vi "计算主体.vi"(2 "算法集合":string[][](array[string])=[["a*(b-c/d)"], ["a-(b-c)+d"], ["a-b+c+d"], ["a*(b+c)-d"], ["a-(b-c)*d"], ["a+b/c+d"], ["a+(b/c)*d"], ["a*b*c-d"], ["a*b+c*d"], ["a*(b+c)+d"], ["a+(b-c)*d"], ["(a-b/c)*d"], ["(a*b-c)*d"], ["(a-(b-c))*d"], ["(a-b+c)*d"], ["a+(b*c)+d"], ["a*b-c*d"], ["(a*(b+c))*d"], ["a*(b-c)-d"], ["(a*(b+c))/d"], ["(a-(b+c))*d"], ["a/(b/c)+d"], ["a/(b-(c/d))"], ["a*(b-c)*d"], ["a*(b-c)+d"], ["a+(b-c)+d"], ["a+(b-c)-d"], ["a+(b*c)-d"], ["(a-(b*c))*d"], ["(a-(b/c))*d"], ["a*b-c*d"], ["a*b+c*d"], ["(a+b/c)*d"], ["b*(a-c/d)"], ["b-(a-c)+d"], ["b-a+c+d"], ["b*(a+c)-d"], ["b-(a-c)*d"], ["b+a/c+d"], ["b+(a/c)*d"], ["b*a*c-d"], ["b*a+c*d"], ["b*(a+c)+d"], ["b+(a-c)*d"], ["(b-a/c)*d"], ["(b*a-c)*d"], ["(b-(a-c))*d"], ["(b-a+c)*d"], ["b+(a*c)+d"], ["b*a-c*d"], ["(b*(a+c))*d"], ["b*(a-c)-d"], ["(b*(a+c))/d"], ["(b-(a+c))*d"], ["b/(a/c)+d"], ["b/(a-(c/d))"], ["b*(a-c)*d"], ["b*(a-c)+d"], ["b+(a-c)+d"], ["b+(a-c)-d"], ["b+(a*c)-d"], ["(b-(a*c))*d"], ["(b-(a/c))*d"], ["b*a-c*d"], ["b*a+c*d"], ["(b+a/c)*d"], ["d*(b-c/a)"], ["d-(b-c)+a"], ["d-b+c+a"], ["d*(b+c)-a"], ["d-(b-c)*a"], ["d+b/c+a"], ["d+(b/c)*a"], ["d*b*c-a"], ["d*b+c*a"], ["d*(b+c)+a"], ["d+(b-c)*a"], ["(d-b/c)*a"], ["(d*b-c)*a"], ["(d-(b-c))*a"], ["(d-b+c)*a"], ["d+(b*c)+a"], ["d*b-c*a"], ["(d*(b+c))*a"], ["d*(b-c)-a"], ["(d*(b+c))/a"], ["(d-(b+c))*a"], ["d/(b/c)+a"], ["d/(b-(c/a))"], ["d*(b-c)*a"], ["d*(b-c)+a"], ["d+(b-c)+a"], ["d+(b-c)-a"], ["d+(b*c)-a"], ["(d-(b*c))*a"], ["(d-(b/c))*a"], ["d*b-c*a"], ["d*b+c*a"], ["(d+b/c)*a"], ["c*(b-a/d)"], ["c-(b-a)+d"], ["c-b+a+d"], ["c*(b+a)-d"], ["c-(b-a)*d"], ["c+b/a+d"], ["c+(b/a)*d"], ["c*b*a-d"], ["c*b+a*d"], ["c*(b+a)+d"], ["c+(b-a)*d"], ["(c-b/a)*d"], ["(c*b-a)*d"], ["(c-(b-a))*d"], ["(c-b+a)*d"], ["c+(b*a)+d"], ["c*b-a*d"], ["(c*(b+a))*d"], ["c*(b-a)-d"], ["(c*(b+a))/d"], ["(c-(b+a))*d"], ["c/(b/a)+d"], ["c/(b-(a/d))"], ["c*(b-a)*d"], ["c*(b-a)+d"], ["c+(b-a)+d"], ["c+(b-a)-d"], ["c+(b*a)-d"], ["(c-(b*a))*d"], ["(c-(b/a))*d"], ["c*b-a*d"], ["c*b+a*d"], ["(c+b/a)*d"], ["a*(b-d/c)"], ["a-(b-d)+c"], ["a-b+d+c"], ["a*(b+d)-c"], ["a-(b-d)*c"], ["a+b/d+c"], ["a+(b/d)*c"], ["a*b*d-c"], ["a*b+d*c"], ["a*(b+d)+c"], ["a+(b-d)*c"], ["(a-b/d)*c"], ["(a*b-d)*c"], ["(a-(b-d))*c"], ["(a-b+d)*c"], ["a+(b*d)+c"], ["a*b-d*c"], ["(a*(b+d))*c"], ["a*(b-d)-c"], ["(a*(b+d))/c"], ["(a-(b+d))*c"], ["a/(b/d)+c"], ["a/(b-(d/c))"], ["a*(b-d)*c"], ["a*(b-d)+c"], ["a+(b-d)+c"], ["a+(b-d)-c"], ["a+(b*d)-c"], ["(a-(b*d))*c"], ["(a-(b/d))*c"], ["a*b-d*c"], ["a*b+d*c"], ["(a+b/d)*c"], ["a*(d-c/b)"], ["a-(d-c)+b"], ["a-d+c+b"], ["a*(d+c)-b"], ["a-(d-c)*b"], ["a+d/c+b"], ["a+(d/c)*b"], ["a*d*c-b"], ["a*d+c*b"], ["a*(d+c)+b"], ["a+(d-c)*b"], ["(a-d/c)*b"], ["(a*d-c)*b"], ["(a-(d-c))*b"], ["(a-d+c)*b"], ["a+(d*c)+b"], ["a*d-c*b"], ["(a*(d+c))*b"], ["a*(d-c)-b"], ["(a*(d+c))/b"], ["(a-(d+c))*b"], ["a/(d/c)+b"], ["a/(d-(c/b))"], ["a*(d-c)*b"], ["a*(d-c)+b"], ["a+(d-c)+b"], ["a+(d-c)-b"], ["a+(d*c)-b"], ["(a-(d*c))*b"], ["(a-(d/c))*b"], ["a*d-c*b"], ["a*d+c*b"], ["(a+d/c)*b"], ["a*(c-b/d)"], ["a-(c-b)+d"], ["a-c+b+d"], ["a*(c+b)-d"], ["a-(c-b)*d"], ["a+c/b+d"], ["a+(c/b)*d"], ["a*c*b-d"], ["a*c+b*d"], ["a*(c+b)+d"], ["a+(c-b)*d"], ["(a-c/b)*d"], ["(a*c-b)*d"], ["(a-(c-b))*d"], ["(a-c+b)*d"], ["a+(c*b)+d"], ["a*c-b*d"], ["(a*(c+b))*d"], ["a*(c-b)-d"], ["(a*(c+b))/d"], ["(a-(c+b))*d"], ["a/(c/b)+d"], ["a/(c-(b/d))"], ["a*(c-b)*d"], ["a*(c-b)+d"], ["a+(c-b)+d"], ["a+(c-b)-d"], ["a+(c*b)-d"], ["(a-(c*b))*d"], ["(a-(c/b))*d"], ["a*c-b*d"], ["a*c+b*d"], ["(a+c/b)*d"], ["a+b+c+d"], ["a*b*c*d"], ["a*b+c+d"], ["a*b+c-d"], ["a*b-c-d"], ["a*b*c+d"], ["a*b*c-d"], ["a*b+c*d"], ["a*b-c*d"], ["a/b+c+d"], ["a+b-c/d"], ["a*b/c+d"], ["a*b/c-d"], ["a*b/c/d"], ["a*b*c/d"], ["a*b+c/d"], ["a*b-c/d"], ["(a+b)*c+d"], ["(a+b)*c-d"], ["(a-b)*c+d"], ["(a-b)*c-d"], ["(a+b)*c*d"], ["(a-b)*c*d"], ["(a+b)*(c+d)"], ["(a-b)*(c-d)"], ["(a-b)*(c+d)"], ["(a+b+c)*d"], ["(a+b-c)*d"], ["(a-b-c)*d"], ["(a*b+c)*d"], ["(a*b-c)*d"], ["(a-b*c)*d"], ["(a*b-c)/d"], ["(a*b+c)/d"], ["a*b/(c+d)"], ["(a+b)/c+d"], ["(a+b)*c/d"], ["(a-b)*c/d"], ["a*b/(c-d)"], ["(c-a*b)*d"], ["b+a+c+d"], ["b*a*c*d"], ["b*a+c+d"], ["b*a+c-d"], ["b*a-c-d"], ["b*a*c+d"], ["b*a*c-d"], ["b*a+c*d"], ["b*a-c*d"], ["b/a+c+d"], ["b+a-c/d"], ["b*a/c+d"], ["b*a/c-d"], ["b*a/c/d"], ["b*a*c/d"], ["b*a+c/d"], ["b*a-c/d"], ["(b+a)*c+d"], ["(b+a)*c-d"], ["(b-a)*c+d"], ["(b-a)*c-d"], ["(b+a)*c*d"], ["(b-a)*c*d"], ["(b+a)*(c+d)"], ["(b-a)*(c-d)"], ["(b-a)*(c+d)"], ["(b+a+c)*d"], ["(b+a-c)*d"], ["(b-a-c)*d"], ["(b*a+c)*d"], ["(b*a-c)*d"], ["(b-a*c)*d"], ["(b*a-c)/d"], ["(b*a+c)/d"], ["b*a/(c+d)"], ["(b+a)/c+d"], ["(b+a)*c/d"], ["(b-a)*c/d"], ["b*a/(c-d)"], ["(c-b*a)*d"], ["c+b+a+d"], ["c*b*a*d"], ["c*b+a+d"], ["c*b+a-d"], ["c*b-a-d"], ["c*b*a+d"], ["c*b*a-d"], ["c*b+a*d"], ["c*b-a*d"], ["c/b+a+d"], ["c+b-a/d"], ["c*b/a+d"], ["c*b/a-d"], ["c*b/a/d"], ["c*b*a/d"], ["c*b+a/d"], ["c*b-a/d"], ["(c+b)*a+d"], ["(c+b)*a-d"], ["(c-b)*a+d"], ["(c-b)*a-d"], ["(c+b)*a*d"], ["(c-b)*a*d"], ["(c+b)*(a+d)"], ["(c-b)*(a-d)"], ["(c-b)*(a+d)"], ["(c+b+a)*d"], ["(c+b-a)*d"], ["(c-b-a)*d"], ["(c*b+a)*d"], ["(c*b-a)*d"], ["(c-b*a)*d"], ["(c*b-a)/d"], ["(c*b+a)/d"], ["c*b/(a+d)"], ["(c+b)/a+d"], ["(c+b)*a/d"], ["(c-b)*a/d"], ["c*b/(a-d)"], ["(a-c*b)*d"], ["d+b+c+a"], ["d*b*c*a"], ["d*b+c+a"], ["d*b+c-a"], ["d*b-c-a"], ["d*b*c+a"], ["d*b*c-a"], ["d*b+c*a"], ["d*b-c*a"], ["d/b+c+a"], ["d+b-c/a"], ["d*b/c+a"], ["d*b/c-a"], ["d*b/c/a"], ["d*b*c/a"], ["d*b+c/a"], ["d*b-c/a"], ["(d+b)*c+a"], ["(d+b)*c-a"], ["(d-b)*c+a"], ["(d-b)*c-a"], ["(d+b)*c*a"], ["(d-b)*c*a"], ["(d+b)*(c+a)"], ["(d-b)*(c-a)"], ["(d-b)*(c+a)"], ["(d+b+c)*a"], ["(d+b-c)*a"], ["(d-b-c)*a"], ["(d*b+c)*a"], ["(d*b-c)*a"], ["(d-b*c)*a"], ["(d*b-c)/a"], ["(d*b+c)/a"], ["d*b/(c+a)"], ["(d+b)/c+a"], ["(d+b)*c/a"], ["(d-b)*c/a"], ["d*b/(c-a)"], ["(c-d*b)*a"], ["a+c+b+d"], ["a*c*b*d"], ["a*c+b+d"], ["a*c+b-d"], ["a*c-b-d"], ["a*c*b+d"], ["a*c*b-d"], ["a*c+b*d"], ["a*c-b*d"], ["a/c+b+d"], ["a+c-b/d"], ["a*c/b+d"], ["a*c/b-d"], ["a*c/b/d"], ["a*c*b/d"], ["a*c+b/d"], ["a*c-b/d"], ["(a+c)*b+d"], ["(a+c)*b-d"], ["(a-c)*b+d"], ["(a-c)*b-d"], ["(a+c)*b*d"], ["(a-c)*b*d"], ["(a+c)*(b+d)"], ["(a-c)*(b-d)"], ["(a-c)*(b+d)"], ["(a+c+b)*d"], ["(a+c-b)*d"], ["(a-c-b)*d"], ["(a*c+b)*d"], ["(a*c-b)*d"], ["(a-c*b)*d"], ["(a*c-b)/d"], ["(a*c+b)/d"], ["a*c/(b+d)"], ["(a+c)/b+d"], ["(a+c)*b/d"], ["(a-c)*b/d"], ["a*c/(b-d)"], ["(b-a*c)*d"], ["a+d+c+b"], ["a*d*c*b"], ["a*d+c+b"], ["a*d+c-b"], ["a*d-c-b"], ["a*d*c+b"], ["a*d*c-b"], ["a*d+c*b"], ["a*d-c*b"], ["a/d+c+b"], ["a+d-c/b"], ["a*d/c+b"], ["a*d/c-b"], ["a*d/c/b"], ["a*d*c/b"], ["a*d+c/b"], ["a*d-c/b"], ["(a+d)*c+b"], ["(a+d)*c-b"], ["(a-d)*c+b"], ["(a-d)*c-b"], ["(a+d)*c*b"], ["(a-d)*c*b"], ["(a+d)*(c+b)"], ["(a-d)*(c-b)"], ["(a-d)*(c+b)"], ["(a+d+c)*b"], ["(a+d-c)*b"], ["(a-d-c)*b"], ["(a*d+c)*b"], ["(a*d-c)*b"], ["(a-d*c)*b"], ["(a*d-c)/b"], ["(a*d+c)/b"], ["a*d/(c+b)"], ["(a+d)/c+b"], ["(a+d)*c/b"], ["(a-d)*c/b"], ["a*d/(c-b)"], ["(c-a*d)*b"], ["a+b+d+c"], ["a*b*d*c"], ["a*b+d+c"], ["a*b+d-c"], ["a*b-d-c"], ["a*b*d+c"], ["a*b*d-c"], ["a*b+d*c"], ["a*b-d*c"], ["a/b+d+c"], ["a+b-d/c"], ["a*b/d+c"], ["a*b/d-c"], ["a*b/d/c"], ["a*b*d/c"], ["a*b+d/c"], ["a*b-d/c"], ["(a+b)*d+c"], ["(a+b)*d-c"], ["(a-b)*d+c"], ["(a-b)*d-c"], ["(a+b)*d*c"], ["(a-b)*d*c"], ["(a+b)*(d+c)"], ["(a-b)*(d-c)"], ["(a-b)*(d+c)"], ["(a+b+d)*c"], ["(a+b-d)*c"], ["(a-b-d)*c"], ["(a*b+d)*c"], ["(a*b-d)*c"], ["(a-b*d)*c"], ["(a*b-d)/c"], ["(a*b+d)/c"], ["a*b/(d+c)"], ["(a+b)/d+c"], ["(a+b)*d/c"], ["(a-b)*d/c"], ["a*b/(d-c)"], ["(d-a*b)*c"], ["((c-a)*b)*d"], ["((c-a)*d)/b"], ["((c-b)*a)*d"], ["((c-b)*d)/a"], ["((b-a)*c)*d"], ["((b-a)*d)/c"], ["((c-a)*d)*b"], ["((c-a)*b)/d"], ["((a-c)*b)*d"], ["((a-c)*d)/b"], ["((d-a)*b)*c"], ["((d-a)*c)/b"], ["((c-d)*b)*a"], ["((c-d)*a)/b"]], 4 "d":dbl, 5 "c":dbl, 6 "b":dbl, 7 "a":dbl) -> (0 "连接的字符串":string, 1 "算法总数":i32, 3 "所有正解":string[](array[string]))   [LabVIEW 2014]
panel:
  out "算法方程":string[][](array[string]) caption="所有行"
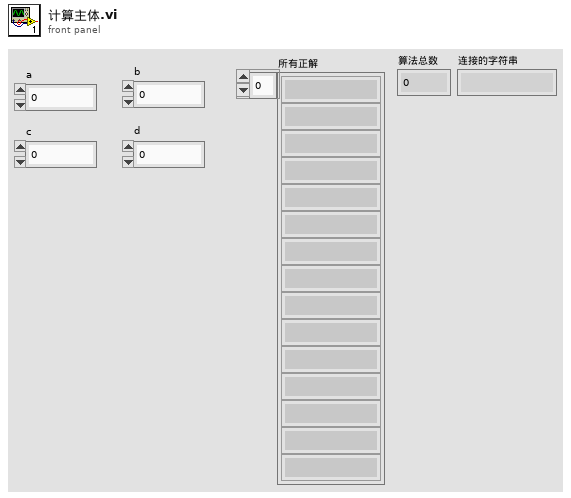
[diagram p1: front panel]
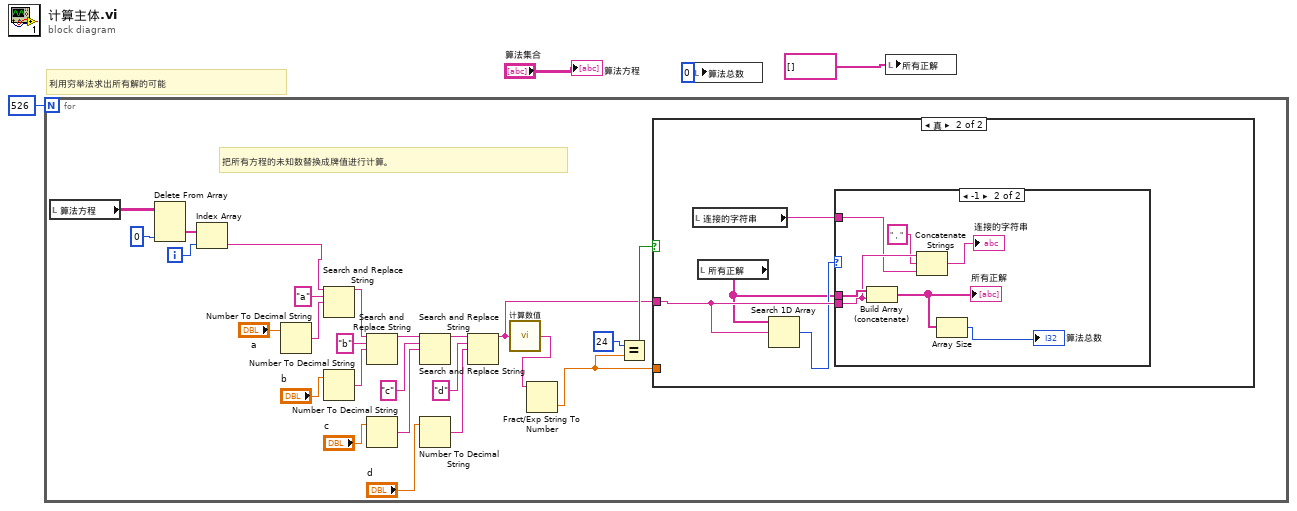
[diagram p0: block diagram]
diagram:
  # "利用穷举法求出所有解的可能"
  n1 = for {
    N: 526 -> [_]
    i -> [w20]
    # "把所有方程的未知数替换成牌值进行计算。"
    n2 = local read "算法方程"() -> (w19:string[][])
    n3 = Delete From Array(array=w19, index (col)=0 ("禁用的索引 (列)")) -> (deleted portion=w21:string[])  [unwired: 2 in, 1 out]
    n4 = Index Array(array=w21, index=w20) -> (element=w7:string)
    n5 = Number To Decimal String(number="a") -> (decimal integer string=w14:string)  [unwired: 1 in]
    n6 = Search and Replace String(input string=w7, search string="a" ("搜索字符串"), replace string=w14) -> (result string=w25:string)  [unwired: 5 in, 3 out]
    n7 = Number To Decimal String(number="b") -> (decimal integer string=w12:string)  [unwired: 1 in]
    n8 = Search and Replace String(input string=w25, search string="b" ("输入字符串"), replace string=w12) -> (result string=w24:string)  [unwired: 5 in, 3 out]
    n9 = Number To Decimal String(number="c") -> (decimal integer string=w10:string)  [unwired: 1 in]
    n10 = Search and Replace String(input string=w24, search string="c" ("输入字符串"), replace string=w10) -> (result string=w23:string)  [unwired: 5 in, 3 out]
    n11 = Number To Decimal String(number="d") -> (decimal integer string=w8:string)  [unwired: 1 in]
    n12 = Search and Replace String(input string=w23, search string="d" ("输入字符串"), replace string=w8) -> (result string=w16:string)  [unwired: 5 in, 3 out]
    n13 = call "计算数值.vi"("表达式"=w16) -> ("结果"=w6:string)
    n14 = Fract/Exp String To Number(string=w6) -> (number=w5:dbl)  [unwired: 3 in, 1 out]
    n15 = Equal?(x=24 ("数字"), y=w5) -> (x = y?=w17:bool)
    n16 = case shown="真" w17 {
      tunnel: w16 -> [_ w33]
      tunnel: w5 -> [_ _]
      frame False {
      }
      frame True {
        n17 = local read "连接的字符串"() -> (w30:string)
        n18 = local read "所有正解"() -> (w31:string[])
        n19 = Search 1D Array(1D array=w31, element=w33) -> (index of element=w32:i32)  [unwired: 1 in]
        n20 = case shown="-1" w32 {
          tunnel: w33 -> [_ w38]
          tunnel: w31 -> [_ w40]
          tunnel: w30 -> [_ w36]
          frame 0, Default {
          }
          frame -1 {
            n21 = Build Array (concatenate)(w40, w38) -> (w39:string[])
            "所有正解" <- w39
            n22 = Concatenate Strings(w38, "，" ("字符串"), w36) -> (→"连接的字符串":string)
            n23 = Array Size(array=w39) -> (size(s)=→"算法总数":i32)
          }
        }
      }
    }
  }
  n24 = local write "算法总数"(0 ("大小")) -> ()
  n25 = local write "所有正解"(string[] [] ("添加的数组")) -> ()
  "算法方程" <- "算法集合"
